vi "Is Error Occured.vi"(8 "error in (no error)":errorcluster, 9 "Enum":enum16{"Get", "Set"}(ring), 11 "Error Occured?":bool) -> (0 "error out":errorcluster, 3 "Error Occured?  2":bool)   [LabVIEW 2017, in "WebServiceImporter.lvlib" / "Error Handling.lvlib"]
uses:
  <vilib>/Platform/WebService/Error Handling/Error Handling.lvlib
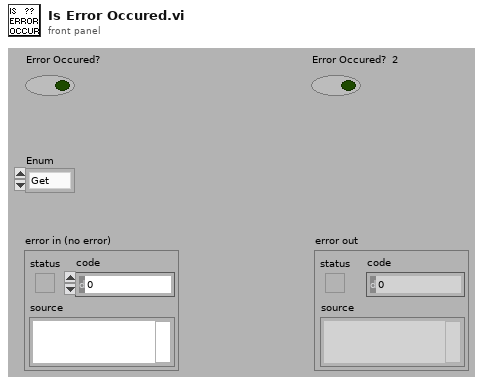
[diagram p1: front panel]
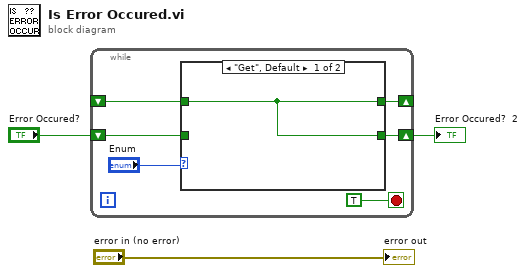
[diagram p0: block diagram]
diagram:
  n1 = while {
    shift-right: [w6] -> w1
    shift-left: "Error Occured?" -> [w7]
    shift-right: [w5] -> _
    shift-left: _ -> [w4]
    stop <- TRUE stop-if-true
    n2 = case shown="\"Get\", Default" "Enum" {
      tunnel: w7 -> [_ w11]
      tunnel: [w10 w11] -> w6
      tunnel: [w10 w11] -> w5
      tunnel: w4 -> [w10 _]
      frame "Get", Default {
      }
      frame "Set" {
      }
    }
  }
  "Error Occured?  2" <- w1
  "error out" <- "error in (no error)"
